vi "Script Methods (XML).vi"(11 "IDM Descriptor Array In":T2) -> (0 "error out":errorcluster, 1 "References to Close":T1(array[cluster]), 2 "Generated XML":string, 3 "IDM Descriptor Array Out":T2, 4 "VIs to Inline":string[](array[string]))   [LabVIEW 2021]
uses:
  <vilib>/myRIO/Common/Express VI Framework/typedefs/Instrument Driver Method Descriptor Array.ctl
  <vilib>/myRIO/Common/Express VI Framework/typedefs/Instrument Driver Method Descriptor.ctl
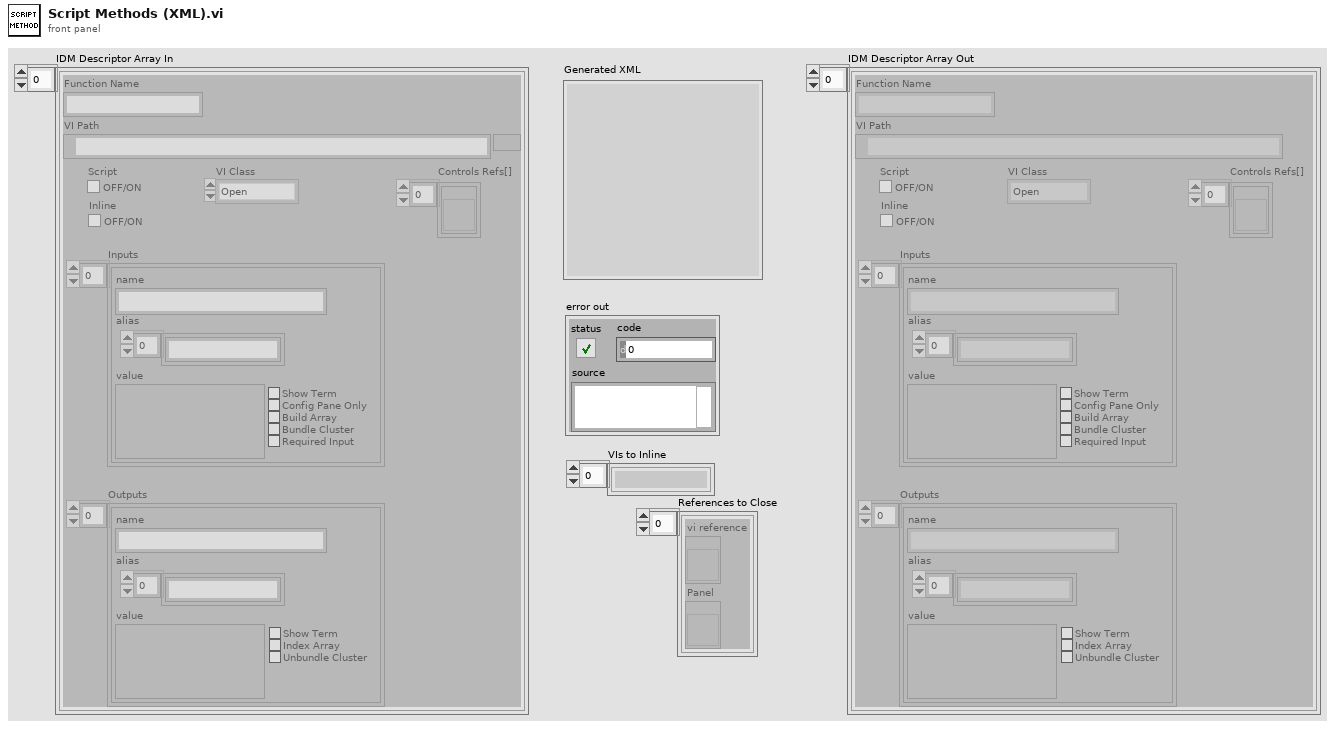
[diagram p1: front panel]
types:
  T1 = cluster{"vi reference":refnum<vi>, "Panel":refnum<vi>}[]
  T2 = typedef "Instrument Driver Method Descriptor Array.ctl" = T3[]
  T3 = typedef "Instrument Driver Method Descriptor.ctl" = cluster{"Function Name":string, "VI Path":path, "Script":bool, "Inputs":cluster{"name":string, "value":variant, "Config Pane Only":bool, "Build Array":bool, "Bundle Cluster":bool, "Show Term":bool, "alias":string[], "Required Input":bool}[], "Outputs":cluster{"name":string, "value":variant, "Show Term":bool, "Index Array":bool, "Unbundle Cluster":bool, "alias":string[]}[], "VI Class":enum16{"Open", "Configure", "Data", "Manage", "Close"}, "Controls Refs[]":refnum<vi>[], "Inline":bool}
  T4 = cluster{"vi reference":refnum<vi>, "Panel":refnum<vi>}
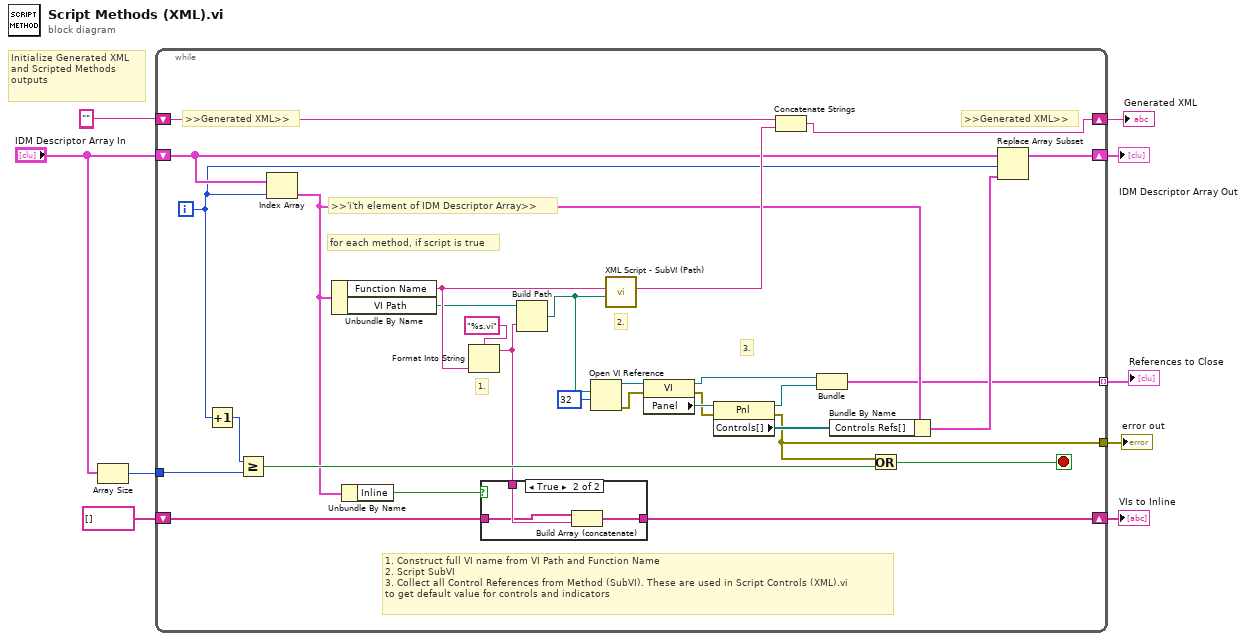
[diagram p0: block diagram]
diagram:
  (unwired) "" ("Generated XML")
  # "Initialize Generated XML and Scripted Methods\noutputs"
  n1 = Array Size(array="IDM Descriptor Array In") -> (size(s)=w7:i32)
  n2 = while {
    shift-right: [w38] -> w5
    shift-left: "" ("Generated XML") -> [w39]
    shift-right: [w21] -> w6
    shift-left: "IDM Descriptor Array In" -> [w24]
    tunnel: w7 -> [w26]
    tunnel: [w19] -> w4
    shift-right: [w14] -> w2
    shift-left: string[] [] ("appended array") -> [w16]
    tunnel: [w11] -> w1 mode=indexing
    i -> [w23]
    stop <- w20 stop-if-true
    # ">>'i'th element of IDM Descriptor Array>>"
    # "1. Construct full VI name from VI Path and Function Name\n2. Script SubVI\n3. Collect all Control References from Method (SubVI). These are used in Script Controls (XML).vi\nto get default value for controls and indicators"
    # "3."
    # "2."
    # "1."
    # "for each method, if script is true"
    # ">>Generated XML>>"
    # ">>Generated XML>>"
    n3 = Increment(x=w23) -> (x+1=w27:i32)
    n4 = Greater Or Equal?(x=w27, y=w26) -> (x >= y?=w25:bool)
    n5 = Index Array(array=w24, index=w23) -> (element=w18:T3)
    n6 = Unbundle By Name(w18) -> ("Function Name"=w37:string, "VI Path"=w35:path)
    n7 = Unbundle By Name(w18) -> ("Inline"=w15:bool)
    n8 = Format Into String(format string="%s.vi", w37) -> (resulting string=w17:string)  [unwired: 2 in, 1 out]
    n9 = case shown="True" w15 {
      tunnel: w17 -> [_ w43]
      tunnel: w16 -> [w40 w42]
      tunnel: [w40 w41] -> w14
      frame False {
      }
      frame True {
        n10 = Build Array (concatenate)(w42, w43) -> (w41:string[])
      }
    }
    n11 = Build Path(base path=w35, name or relative path=w17) -> (appended path=w33:path)
    n12 = Open VI Reference(vi path=w33, options=32) -> (vi reference=w32:refnum<vi>, error out=w30:errorcluster)  [unwired: 4 in]
    n13 = call <vilib>:"XML Script - SubVI (Path).vi"("path"=w33, "name"=w37) -> ("XML Script Command - SubVI"=w34:string)  [unwired: 8 in, 1 out]
    n14 = property class="VI"(reference=w32, error in=w30) -> (reference out=w13:refnum<vi>, error out=w29:errorcluster, "Panel"=w31:refnum<vi>)
    n15 = property class="Pnl"(reference=w31, error in=w29) -> (reference out=w12:refnum<vi>, error out=w19:errorcluster, "Controls[]"=w28:refnum<vi>[])
    n16 = Concatenate Strings(w39, w34) -> (w38:string)
    n17 = Bundle("vi reference"=w13, "Panel"=w12) -> (w11:T4)  [unwired: 1 in]
    n18 = Bundle By Name(cluster=w18, "Controls Refs[]"=w28) -> (w22:T3)
    n19 = Or(x=w19, y=w25) -> (x .or. y?=w20:bool)
    n20 = Replace Array Subset(array=w24, new element=w22, index=w23) -> (w21:T2)
  }
  "Generated XML" <- w5
  "IDM Descriptor Array Out" <- w6
  "error out" <- w4
  "VIs to Inline" <- w2
  "References to Close" <- w1
